vi "test String to U8_1.vi"(11 "Test Case In":refnum<class "test Electronic Datasheet.lvclass">) -> (0 "error out":errorcluster, 3 "Test Case Out":refnum<class "test Electronic Datasheet.lvclass">)   [LabVIEW 2024, in "Test Utilities.lvclass"]
uses:
  Test Utilities.lvclass
  Test Utilities.lvclass/Test Utilities.ctl
  EDS-File-Viewer/Tests/source/test Electronic Datasheet/test Electronic Datasheet.lvclass
  <vilib>/Astemes/LUnit/Test Case.lvclass
  source/CANopen.lvlib
panel:
  out "Byte":u8
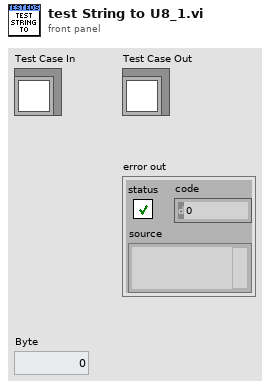
[diagram p1: front panel]
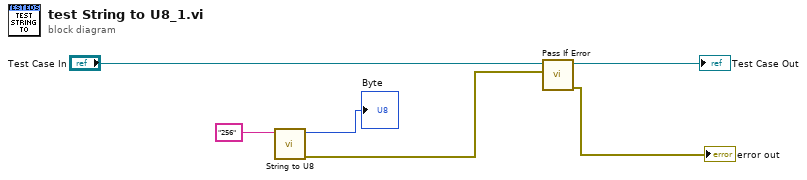
[diagram p0: block diagram]
diagram:
  n1 = call "String to U8.vi"("Integer String"="256" ("String")) -> ("error out"=w2:errorcluster, "U8"=→"Byte":u8)  [unwired: 9 in]
  n2 = call <vilib>:"Pass If Error.vi"("Assert error"=w2, "LUnit Test Case In"="Test Case In") -> ("error out"=→"error out":errorcluster, "LUnit Test Case Out"=→"Test Case Out":refnum<class "test Electronic Datasheet.lvclass">)  [unwired: 8 in]
